vi "FuncImg-Event handler-Z plane value change.vi"() -> ()   [LabVIEW 2013]
uses:
  Global variables/gl_Functional Imaging-Global variables.vi
panel:
  out "error out":errorcluster
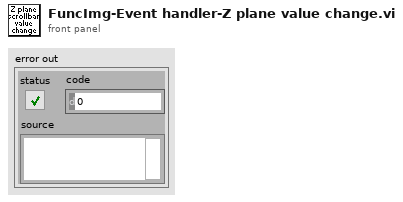
[diagram p1: front panel]
types:
  T1 = typedef "Functional Imging UI Refs.ctl" = cluster{"Menu ref":refnum<k9>, "Image control":refnum<vi>, "VI ref":refnum<vi>, "XGrapher":refnum<vi>, "Smoothing":refnum<vi>, "POI Averaging":refnum<vi>, "Normalize":refnum<vi>, "POI data points in each trial":refnum<vi>, "Channel":refnum<vi>, "Experiment data folder path":refnum<vi>, "[ROI vis]":refnum<vi>, "[Groups] visbl":T2, "Group Name":refnum<vi>, "POI index":refnum<vi>, "Trial No.":refnum<vi>, "Intensity Zoom":refnum<vi>, "Trial Cursor Enabled":refnum<vi>, "Number of Trials (ind 1)":refnum<vi>, "Number of Trials (ind 2)":refnum<vi>, "MiniScans Available":refnum<vi>, "POI Available":refnum<vi>, "Defer graph updates":refnum<vi>, "Waveform selector":refnum<vi>, "#of selected POI":refnum<vi>, "#of selected MiniScans":refnum<vi>, "#of selected groups":refnum<vi>, "Max Z-Projection":refnum<vi>, "Z-Plane Selector":refnum<vi>, "Index of miniscan point to visualise":refnum<vi>, "ROI vis. mode":refnum<vi>, "Total # of points":refnum<vi>, "Index of group clicked on":refnum<vi>, "Pane 1":refnum<vi>, "Pane 2":refnum<vi>, "Pane 3":refnum<vi>, "Pane 4":refnum<vi>, "Pane 5":refnum<vi>, "Pane 6":refnum<vi>, "Deselect all ROI":refnum<vi>, "Deselect all groups":refnum<vi>}
  T2 = typedef "Groups array referecne.ctl" = refnum<vi>
  T3 = typedef "IMAQ Image.ctl" = refnum<image>
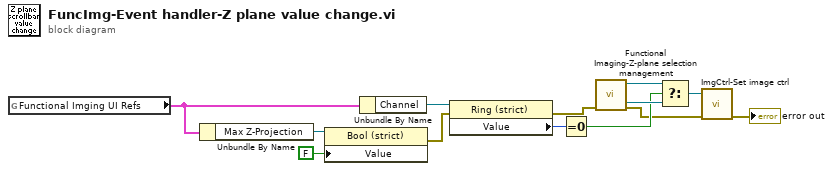
[diagram p0: block diagram]
diagram:
  n1 = global read "gl_Functional Imaging-Global variables.vi" "Functional Imging UI Refs"() -> (w13:T1)
  n2 = Unbundle By Name(w13) -> ("Max Z-Projection"=w9:refnum<vi>)
  n3 = property class="Bool (strict)"(reference=w9, "Value"=FALSE) -> (error out=w2:errorcluster)  [unwired: 1 in, 1 out]
  n4 = Unbundle By Name(w13) -> ("Channel"=w6:refnum<vi>)
  n5 = property class="Ring (strict)"(reference=w6, error in=w2) -> (error out=w3:errorcluster, "Value"=w5:u16)  [unwired: 1 out]
  n6 = Equal To 0?(x=w5) -> (x = 0?=w7:bool)
  n7 = call "Functional Imaging-Z-plane selection management.vi"("error in"=w3) -> ("error out"=w4:errorcluster, "GreenPOIMax"=w11:T3, "RedPOIMax"=w8:T3)  [unwired: 8 in]
  n8 = Select(t=w8, s=w7, f=w11) -> (s? t:f=w12:T3)
  n9 = call "ImgCtrl-Set image ctrl.vi"("error in"=w4, "Image"=w12) -> ("error out"=→"error out":errorcluster)  [unwired: 9 in]
